vi "Get Test Instance Name.vi"(9 "Class Name":string, 10 "LabVIEW Object":refnum<class>) -> (1 "Instance Name":string)   [LabVIEW 2013, in "GraphicalTestRunner.lvlib"]
doc: "Returns the instance name for this Test Case object.\n\nIf the input object is not a Test Case object, Instance Name out = Class Name.\nIf the input Test Case object has not been assigned an instance name, Instance Name out = Class Name."
uses:
  GraphicalTestRunner.lvlib
  Classes/TestCase/TestCase.lvclass
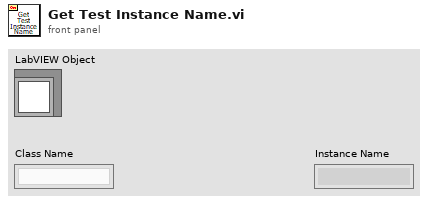
[diagram p1: front panel]
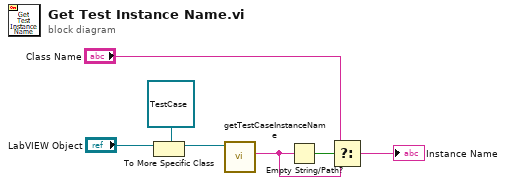
[diagram p0: block diagram]
diagram:
  n1 = To More Specific Class(target class=refnum<class "TestCase.lvclass"> refnum ("TestCase.lvclass"), reference="LabVIEW Object") -> (specific class reference=w5:refnum<class "TestCase.lvclass">)  [unwired: 1 in, 1 out]
  n2 = call "getTestCaseInstanceName.vi"("TestCase in"=w5) -> ("Test Case Instance Name"=w2:string)  [unwired: 9 in, 1 out]
  n3 = Empty String/Path?(string/path=w2) -> (empty?=w4:bool)
  n4 = Select(t="Class Name", s=w4, f=w2) -> (s? t:f=→"Instance Name":string)
